vi "Get Button A.vi"(8 "error in (no error)":errorcluster) -> (0 "error out":errorcluster, 3 "A Pressed":bool)   [LabVIEW 2015]
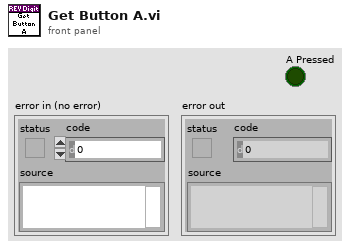
[diagram p1: front panel]
types:
  T1 = typedef "WPI_DigitalInputDevRef.ctl" = cluster{"DevStatus":errorcluster, "DIO Channel":T2}
  T2 = typedef "FPGA_DIOChannel.ctl" = enum8{"DIO 0", "DIO 1", "DIO 2", "DIO 3", "DIO 4", "DIO 5", "DIO 6", "DIO 7", "DIO 8", "DIO 9", "DIO MXP 0", "DIO MXP 1", "DIO MXP 2", "DIO MXP 3", "DIO MXP 4", "DIO MXP 5", "DIO MXP 6", "DIO MXP 7", "DIO MXP 8", "DIO MXP 9", "DIO MXP 10", "DIO MXP 11", "DIO MXP 12", "DIO MXP 13", "DIO MXP 14", "DIO MXP 15", "Invalid"}
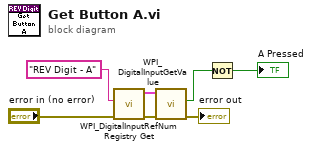
[diagram p0: block diagram]
diagram:
  n1 = call <vilib>:"WPI_DigitalInputRefNum Registry Get.vi"("error in (no error)"="error in (no error)", "refnum name"="REV Digit - A") -> ("error out"=w4:errorcluster, "DigitalInputDevRef"=w6:T1)  [unwired: 8 in]
  n2 = call <vilib>:"WPI_DigitalInputGetValue.vi"("error in (no error)"=w4, "DigitalInputDevRef"=w6) -> ("error out"=→"error out":errorcluster, "Value"=w2:bool)  [unwired: 7 in, 1 out]
  n3 = Not(x=w2) -> (.not. x?=→"A Pressed":bool)
